vi "Display Data.vi"(8 "error in (no error)":errorcluster, 10 "Graph Data":waveform(dbl)[](array[waveform]), 11 "Acquisition UI in":refnum<class "Acquisition UI.lvclass">) -> (0 "error out":errorcluster, 3 "Acquisition UI out":refnum<class "Acquisition UI.lvclass">)   [LabVIEW 2018, in "Acquisition UI.lvlib" / "Acquisition UI.lvclass"]
uses:
  Acquisition UI.lvclass
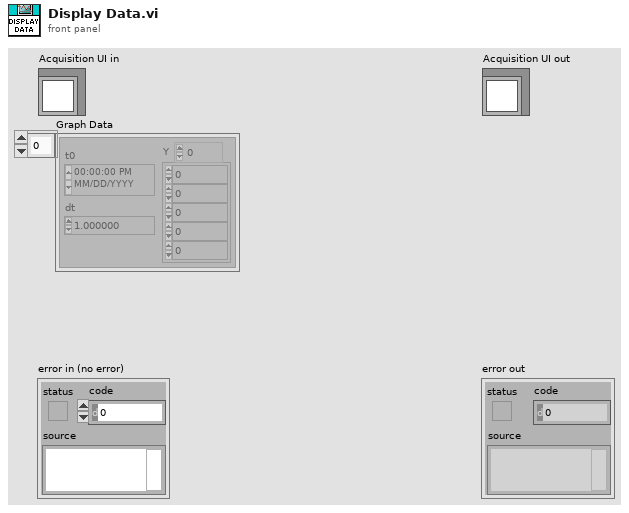
[diagram p1: front panel]
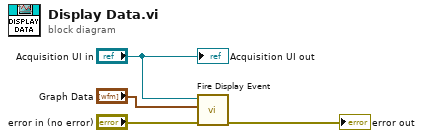
[diagram p0: block diagram]
diagram:
  n1 = call "Fire Display Event.vi"("error in (no error)"="error in (no error)", "Graph Data"="Graph Data", "Acquisition UI in"="Acquisition UI in") -> ("error out"=→"error out":errorcluster)  [unwired: 7 in, 1 out]
  "Acquisition UI out" <- "Acquisition UI in"
